vi "Fire User Event - ConnectionEvent.vi"(8 "error in (no error)":errorcluster, 10 "ConnectionInfo":T1, 11 "ConnectionEvent":refnum<user-event>) -> (0 "error out":errorcluster)   [LabVIEW 2022 SP3, in "User Event - ConnectionEvent.lvlib"]
doc: "Send the Stop event to stop the Event Handling Loop."
uses:
  User Event - ConnectionEvent.lvlib
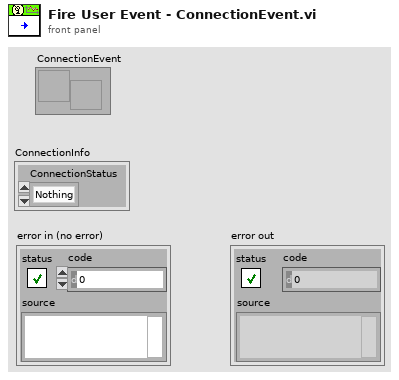
[diagram p1: front panel]
types:
  T1 = cluster{"ConnectionStatus":enum16{"Nothing", "Disconnect", "Connect", "Error"}}
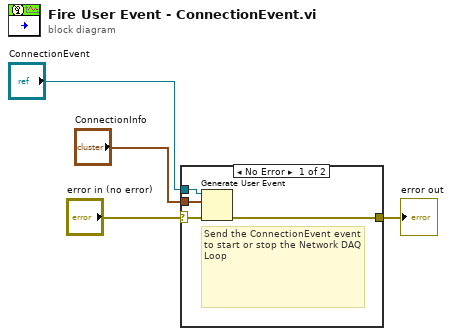
[diagram p0: block diagram]
diagram:
  n1 = case shown="No Error" "error in (no error)" {
    selector: "error in (no error)" -> [w7 w9]
    tunnel: [w8 w9] -> w4
    tunnel: "ConnectionEvent" -> [w6 _]
    tunnel: "ConnectionInfo" -> [w5 _]
    frame No Error {
      # "Send the ConnectionEvent event to start or stop the Network DAQ Loop"
      n2 = Generate User Event(user event=w6, event data cluster=w5, error in=w7) -> (error out=w8:errorcluster)  [unwired: 1 in, 1 out]
    }
    frame Error {
    }
  }
  "error out" <- w4
